vi "wb6PlanMacro.vi"(7 "TargetQty":string="400", 8 "error in (no error)":errorcluster, 10 "Days":i32, 11 "report in":refnum<class "NI_report.lvclass">) -> (0 "error out":errorcluster, 3 "report out":refnum<class "NI_report.lvclass">)   [LabVIEW 2012]
uses:
  <vilib>/Utility/NIReport.llb/NI_report.lvclass
  <vilib>/Utility/NIReport.llb/Excel/NI_Excel.lvclass
  <vilib>/addons/_office/NI_ReportGenerationToolkit.lvlib
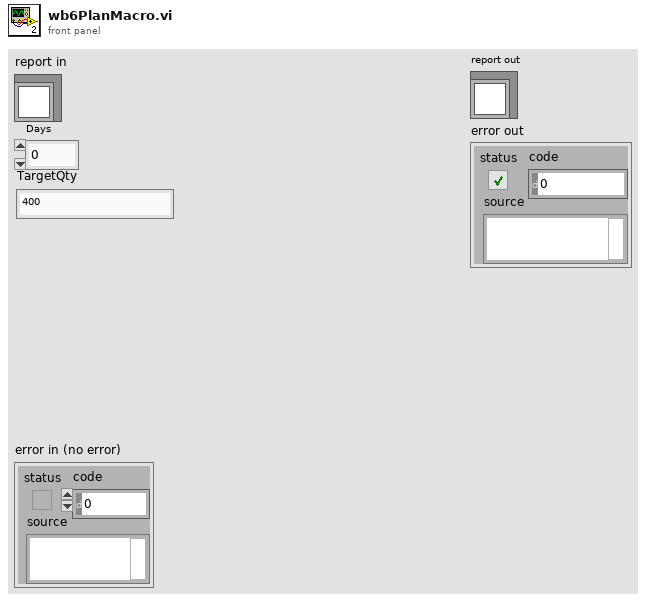
[diagram p1: front panel]
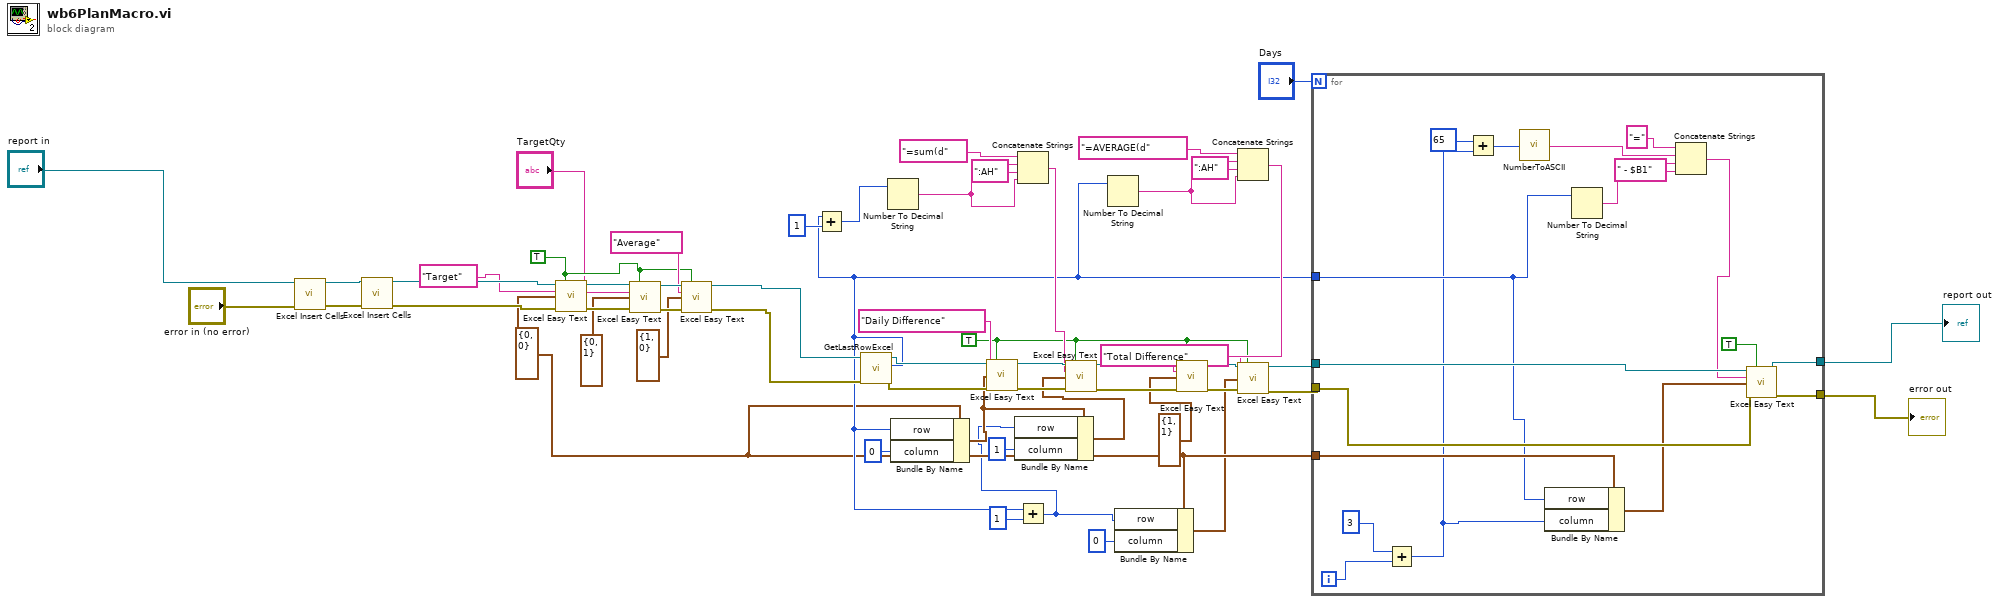
[diagram p0: block diagram]
diagram:
  w14 = TRUE ("border? (F)")
  w43 = TRUE ("border? (F)")
  w9 = cluster{"row":i32, "column":i32} {"row"=0, "column"=0} ("end (-1, -1)")
  n1 = call <vilib>:"Excel Insert Cells.vi"("report in"="report in", "error in (no error)"="error in (no error)") -> ("report out"=w53:refnum<class "NI_report.lvclass">, "error out"=w52:errorcluster)  [unwired: 12 in]
  n2 = call <vilib>:"Excel Insert Cells.vi"("report in"=w53, "error in (no error)"=w52) -> ("report out"=w55:refnum<class "NI_report.lvclass">, "error out"=w54:errorcluster)  [unwired: 12 in]
  n3 = call <vilib>:"Excel Easy Text.vi"("report in"=w55, "border? (F)"=w43, "text"="Target", "start (-1, -1)"=w9, "error in (no error)"=w54) -> ("report out"=w50:refnum<class "NI_report.lvclass">, "error out"=w49:errorcluster)  [unwired: 6 in, 3 out]
  n4 = call <vilib>:"Excel Easy Text.vi"("report in"=w50, "border? (F)"=w43, "text"="TargetQty", "start (-1, -1)"=cluster{"row":i32, "column":i32} {"row"=0, "column"=1} ("end (-1, -1)"), "error in (no error)"=w49) -> ("report out"=w47:refnum<class "NI_report.lvclass">, "error out"=w46:errorcluster)  [unwired: 6 in, 3 out]
  n5 = call <vilib>:"Excel Easy Text.vi"("report in"=w47, "border? (F)"=w43, "text"="Average", "start (-1, -1)"=cluster{"row":i32, "column":i32} {"row"=1, "column"=0} ("end (-1, -1)"), "error in (no error)"=w46) -> ("report out"=w24:refnum<class "NI_report.lvclass">, "error out"=w23:errorcluster)  [unwired: 6 in, 3 out]
  n6 = call "GetLastRowExcel.vi"("error in (no error)"=w23, "report in"=w24) -> ("error out"=w40:errorcluster, "row"=w12:i32, "report out"=w41:refnum<class "NI_report.lvclass">)  [unwired: 7 in]
  n7 = Add(x=w12, y=1) -> (x+y=w29:i32)
  n8 = Number To Decimal String(number=w29) -> (decimal integer string=w32:string)  [unwired: 1 in]
  n9 = Bundle By Name(cluster=w9, "row"=w12, "column"=0) -> (w36:cluster{"row":i32, "column":i32})
  n10 = call <vilib>:"Excel Easy Text.vi"("report in"=w41, "border? (F)"=w14, "text"="Daily Difference", "start (-1, -1)"=w36, "error in (no error)"=w40) -> ("report out"=w31:refnum<class "NI_report.lvclass">, "error out"=w38:errorcluster)  [unwired: 6 in, 3 out]
  n11 = Concatenate Strings("=sum(d" ("string"), w32, ":AH" ("string"), w32) -> (w30:string)
  n12 = Add(x=w12, y=1) -> (x+y=w7:i32)
  n13 = Bundle By Name(cluster=w36, "row"=w7, "column"=1) -> (w35:cluster{"row":i32, "column":i32})
  n14 = call <vilib>:"Excel Easy Text.vi"("report in"=w31, "border? (F)"=w14, "text"=w30, "start (-1, -1)"=w35, "error in (no error)"=w38) -> ("report out"=w22:refnum<class "NI_report.lvclass">, "error out"=w21:errorcluster)  [unwired: 6 in, 3 out]
  n15 = Number To Decimal String(number=w12) -> (decimal integer string=w25:string)  [unwired: 1 in]
  n16 = Bundle By Name(cluster=w9, "row"=w7, "column"=0) -> (w8:cluster{"row":i32, "column":i32})
  n17 = Concatenate Strings("=AVERAGE(d" ("string"), w25, ":AH" ("string"), w25) -> (w19:string)
  n18 = call <vilib>:"Excel Easy Text.vi"("report in"=w22, "border? (F)"=w14, "text"=w19, "start (-1, -1)"=cluster{"row":i32, "column":i32} {"row"=1, "column"=1} ("end (-1, -1)"), "error in (no error)"=w21) -> ("report out"=w18:refnum<class "NI_report.lvclass">, "error out"=w16:errorcluster)  [unwired: 6 in, 3 out]
  n19 = call <vilib>:"Excel Easy Text.vi"("report in"=w18, "border? (F)"=w14, "text"="Total Difference", "start (-1, -1)"=w8, "error in (no error)"=w16) -> ("report out"=w17:refnum<class "NI_report.lvclass">, "error out"=w15:errorcluster)  [unwired: 6 in, 3 out]
  n20 = for {
    N: "Days" -> [_]
    tunnel: w9 -> [w73]
    tunnel: w17 -> [w72]
    tunnel: w15 -> [w71]
    tunnel: [w70] -> w4
    tunnel: [w69] -> w3
    tunnel: w12 -> [w66]
    i -> [w57]
    n21 = Add(x=3 ("column"), y=w57) -> (x+y=w56:i32)
    n22 = Add(x=65, y=w56) -> (x+y=w60:i32)
    n23 = call "NumberToASCII.vi"("number"=w60) -> ("ASCII"=w59:string)
    n24 = Bundle By Name(cluster=w73, "row"=w66, "column"=w56) -> (w68:cluster{"row":i32, "column":i32})
    n25 = Number To Decimal String(number=w66) -> (decimal integer string=w65:string)  [unwired: 1 in]
    n26 = Concatenate Strings("=" ("string"), w59, w65, " - $B1" ("string")) -> (w63:string)
    n27 = call <vilib>:"Excel Easy Text.vi"("report in"=w72, "border? (F)"=TRUE, "text"=w63, "start (-1, -1)"=w68, "error in (no error)"=w71) -> ("report out"=w70:refnum<class "NI_report.lvclass">, "error out"=w69:errorcluster)  [unwired: 6 in, 3 out]
  }
  "report out" <- w4
  "error out" <- w3
